vi "_emi_ SMLoop Error Check.vi"(0 "Loop Index":u16, 1 "Command ID":T1, 7 "Loop  Current Error State":errorcluster, 9 "Current Loop Error/Warning Source":enum16{"No Error", "Start", "Normal", "Stop"}(ring), 11 "Error in":errorcluster) -> (4 "Loop Index out":u16, 8 "Loop Error state out":errorcluster, 10 "Source Out":enum16{"No Error", "Start", "Normal", "Stop"}(ring), 15 "error out":errorcluster)   [LabVIEW 2011]
uses:
  _emi_ SMLoop sates.ctl
  emi_Read System ID.vi
  Private/_emi_GFV System ID.vi
  <vilib>/Utility/error.llb/Clear Errors.vi
  S&E reporting/Private/_emi_S&E Q Generator.vi
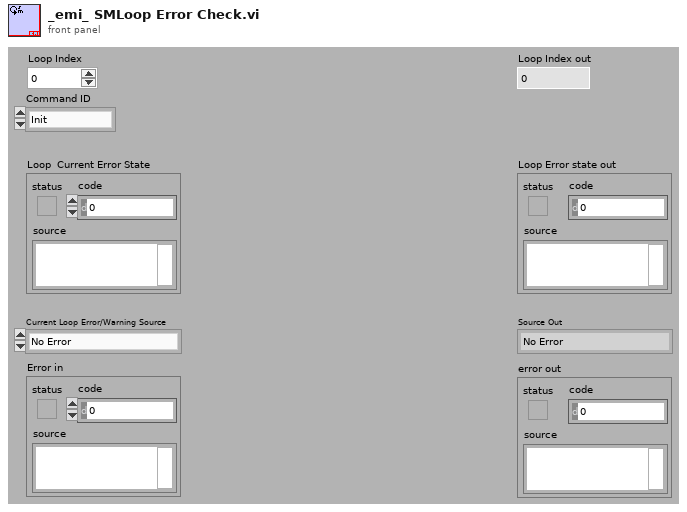
[diagram p1: front panel]
types:
  T1 = typedef "_emi_ SMLoop sates.ctl" = enum16{"Init", "Standby", "Start", "Normal Operation", "Stop", "Error Handling", "End", "Post"}
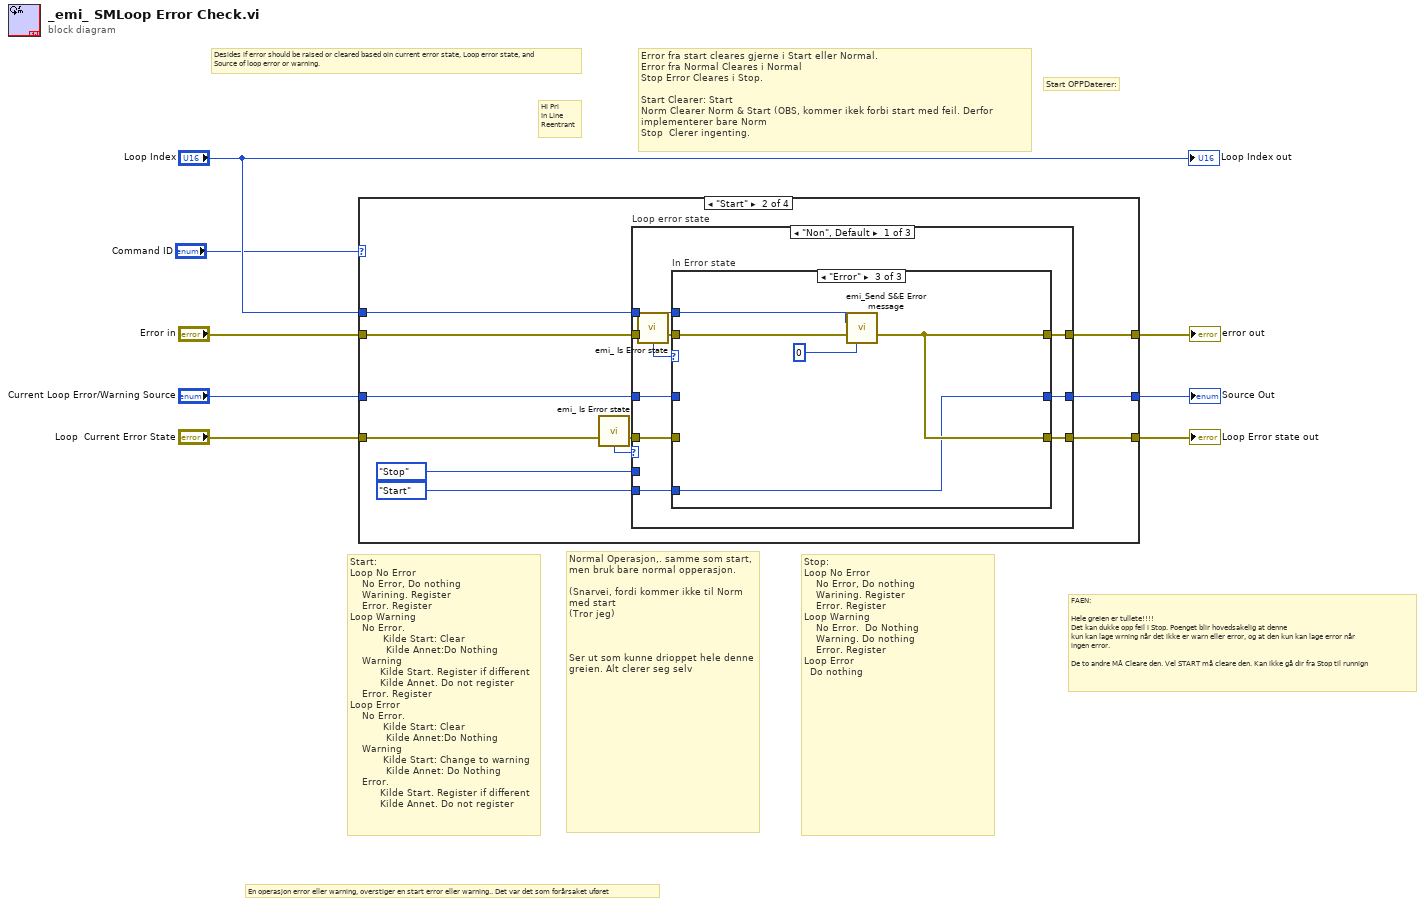
[diagram p0: block diagram]
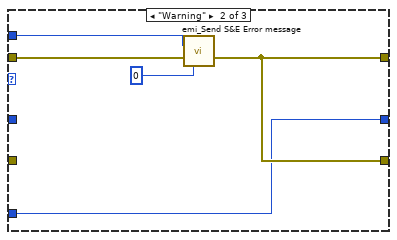
[diagram p4: hidden frame]
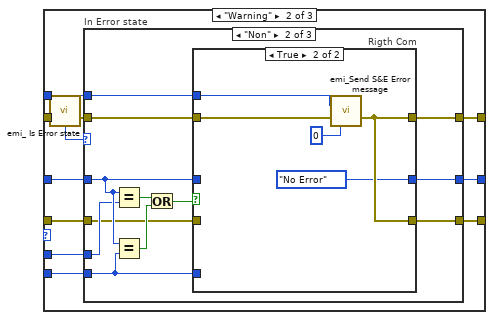
[diagram p5: hidden frame]
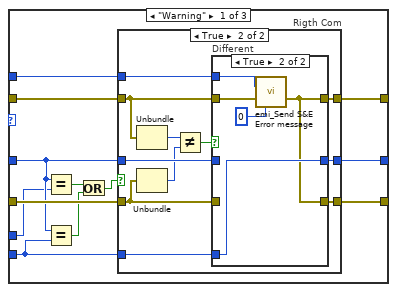
[diagram p6: hidden frame]
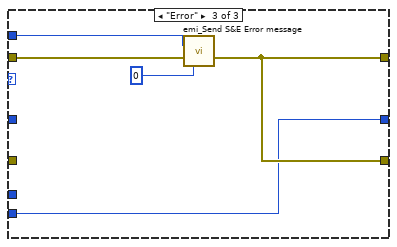
[diagram p10: hidden frame]
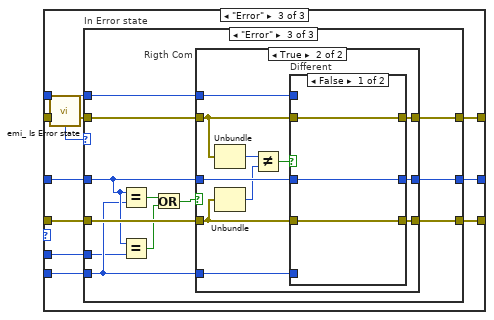
[diagram p11: hidden frame]
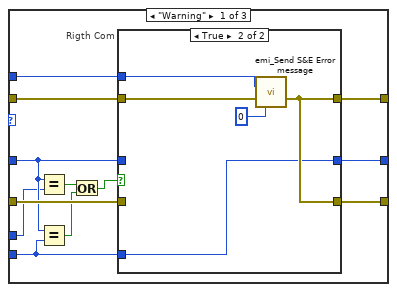
[diagram p12: hidden frame]
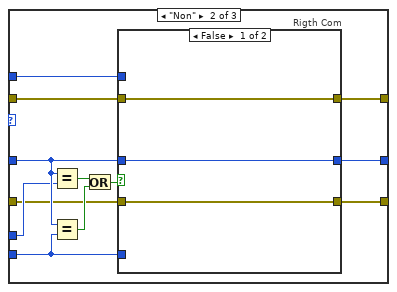
[diagram p14: hidden frame]
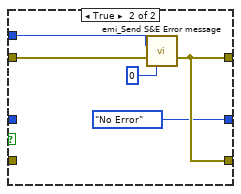
[diagram p15: hidden frame]
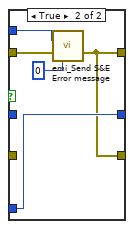
[diagram p17: hidden frame]
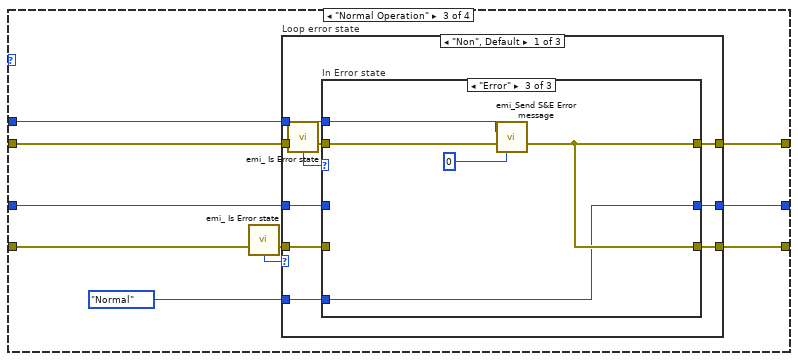
[diagram p18: hidden frame]
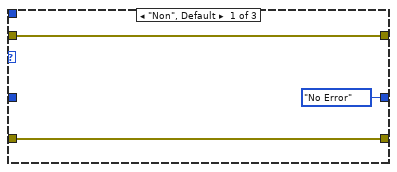
[diagram p19: hidden frame]
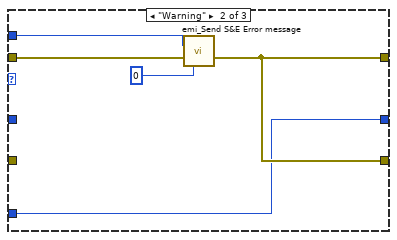
[diagram p20: hidden frame]
diagram:
  # "FAEN:\n\nHele greien er tullete!!!!\nDet kan dukke opp feil i Stop. Poenget blir hovedsakelig at denne\nkun kan lage wrning når det ikke er warn eller error, og at den kun kan lage error når\ningen error.\n\nDe to andre MÅ Cleare den. Vel START må cleare den. Kan ikke gå dir fra Stop til runnign"
  # "Stop:\nLoop No Error          \n    No Error, Do nothing\n    Warining. Register\n    Error. Register\nLoop Warning\n    No Error.  Do Nothing\n    Warning. Do nothing\n    Error. Register\nLoop Error\n  Do nothing"
  # "Normal Operasjon,. samme som start, men bruk bare normal opperasjon.\n\n(Snarvei, fordi kommer ikke til Norm med start\n(Tror jeg)\n\n\n\nSer ut som kunne drioppet hele denne greien. Alt clerer seg selv"
  # "En operasjon error eller warning, overstiger en start error eller warning.. Det var det som forårsaket uføret"
  # "Start OPPDaterer:"
  # "Start:\nLoop No Error          \n    No Error, Do nothing\n    Warining. Register\n    Error. Register\nLoop Warning\n    No Error. \n           Kilde Start: Clear\n            Kilde Annet:Do Nothing\n    Warning\n          Kilde Start. Register if different\n          Kilde Annet. Do not register\n    Error. Register\nLoop Error\n    No Error. \n           Kilde Start: Clear\n            Kilde Annet:Do Nothing\n    Warning\n           Kilde Start: Change to warning\n            Kilde Annet: Do Nothing\n    Error.\n          Kilde Start. Register if different\n          Kilde Annet. Do not register"
  # "Error fra start cleares gjerne i Start eller Normal.\nError fra Normal Cleares i Normal\nStop Error Cleares i Stop.\n\nStart Clearer: Start\nNorm Clearer Norm & Start (OBS, kommer ikek forbi start med feil. Derfor implementerer bare Norm\nStop  Clerer ingenting."
  # "Desides if error should be raised or cleared based oin current error state, Loop error state, and \nSource of loop error or warning."
  # "Hi Pri \nIn Line \nReentrant"
  n1 = case shown="\"Start\"" "Command ID" {
    tunnel: "Loop  Current Error State" -> [w9 w18 w206 w317]
    tunnel: [w9 w22 w210 w321] -> w7
    tunnel: [w10 w21 w209 w320] -> w6
    tunnel: "Current Loop Error/Warning Source" -> [w10 w13 w201 w312]
    tunnel: [w11 w20 w208 w319] -> w4
    tunnel: "Error in" -> [w11 w15 w203 w314]
    tunnel: "Loop Index" -> [_ w19 w207 w318]
    frame "Init", Default {
    }
    frame "Start" {
      n2 = call "emi_ Is Error state.vi"("error in (no error)"=w18) -> ("error out"=w17:errorcluster, "Error State"=w16:enum16{"Non", "Warning", "Error"})  [unwired: 13 in]
      n3 = case "Loop error state" shown="\"Non\", Default" w16 {
        tunnel: w19 -> [w32 w56 w126]
        tunnel: [w31 w55 w125] -> w20
        tunnel: w13 -> [w29 w53 w123]
        tunnel: [w30 w54 w124] -> w21
        tunnel: [w28 w52 w122] -> w22
        tunnel: w17 -> [w27 w51 w121]
        tunnel: w15 -> [w26 w50 w120]
        tunnel: enum16{"No Error", "Start", "Normal", "Stop"}."Start" ("Error source") -> [w23 w47 w117]
        tunnel: enum16{"No Error", "Start", "Normal", "Stop"}."Stop" ("Error source") -> [_ w46 w116]
        frame "Non", Default {
          n4 = call "emi_ Is Error state.vi"("error in (no error)"=w26) -> ("error out"=w25:errorcluster, "Error State"=w24:enum16{"Non", "Warning", "Error"})  [unwired: 13 in]
          n5 = case "In Error state" shown="\"Error\"" w24 {
            tunnel: w32 -> [_ w40 w45]
            tunnel: [w34 w37 w42] -> w31
            tunnel: w25 -> [w34 w38 w43]
            tunnel: [w35 w36 w41] -> w30
            tunnel: w29 -> [w35 _ _]
            tunnel: [w33 w37 w42] -> w28
            tunnel: w27 -> [w33 _ _]
            tunnel: w23 -> [_ w36 w41]
            frame "Non", Default {
            }
            frame "Warning" {
              n6 = call "emi_Send S&E Error message.vi"("Loop ID in(No Loop)"=w40, "error in (no error)"=w38, "Var Index"=u16 0 ("Loc Sub ID")) -> ("error out"=w37:errorcluster)  [unwired: 11 in, 1 out]
            }
            frame "Error" {
              n7 = call "emi_Send S&E Error message.vi"("Loop ID in(No Loop)"=w45, "error in (no error)"=w43, "Var Index"=u16 0 ("Loc Sub ID")) -> ("error out"=w42:errorcluster)  [unwired: 11 in, 1 out]
            }
          }
        }
        frame "Warning" {
          n8 = call "emi_ Is Error state.vi"("error in (no error)"=w50) -> ("error out"=w49:errorcluster, "Error State"=w48:enum16{"Non", "Warning", "Error"})  [unwired: 13 in]
          n9 = case "In Error state" shown="\"Non\"" w48 {
            tunnel: w56 -> [w68 w102 w115]
            tunnel: [w67 w101 w112] -> w55
            tunnel: w49 -> [w64 w98 w113]
            tunnel: [w65 w99 w111] -> w54
            tunnel: w53 -> [w59 w94 _]
            tunnel: [w66 w100 w112] -> w52
            tunnel: w51 -> [w63 w91 _]
            tunnel: w47 -> [w58 w93 w111]
            tunnel: w46 -> [w57 w92 _]
            frame "Warning" {
              n10 = Equal?(x=w59, y=w57) -> (x = y?=w62:bool)
              n11 = Equal?(x=w59, y=w58) -> (x = y?=w61:bool)
              n12 = Or(x=w62, y=w61) -> (x .or. y?=w60:bool)
              n13 = case "Rigth Com" shown="True" w60 {
                tunnel: w68 -> [_ w82]
                tunnel: w64 -> [w70 w80]
                tunnel: [w70 w81] -> w67
                tunnel: [w71 w79] -> w66
                tunnel: [w69 w78] -> w65
                tunnel: w58 -> [_ w72]
                tunnel: w63 -> [w71 w76]
                tunnel: w59 -> [w69 w77]
                frame False {
                }
                frame True {
                  n14 = Unbundle(w80) -> ("code"=w75:i32)  [unwired: 2 out]
                  n15 = Unbundle(w76) -> ("code"=w74:i32)  [unwired: 2 out]
                  n16 = Not Equal?(x=w75, y=w74) -> (x != y?=w73:bool)
                  n17 = case "Different" shown="True" w73 {
                    tunnel: w82 -> [_ w90]
                    tunnel: w80 -> [w84 w88]
                    tunnel: [w84 w86] -> w81
                    tunnel: w76 -> [w85 _]
                    tunnel: [w85 w86] -> w79
                    tunnel: [w83 w87] -> w78
                    tunnel: w77 -> [w83 _]
                    tunnel: w72 -> [_ w87]
                    frame False {
                    }
                    frame True {
                      n18 = call "emi_Send S&E Error message.vi"("Loop ID in(No Loop)"=w90, "error in (no error)"=w88, "Var Index"=u16 0 ("Loc Sub ID")) -> ("error out"=w86:errorcluster)  [unwired: 11 in, 1 out]
                    }
                  }
                }
              }
            }
            frame "Non" {
              n19 = Equal?(x=w94, y=w92) -> (x = y?=w97:bool)
              n20 = Equal?(x=w94, y=w93) -> (x = y?=w96:bool)
              n21 = Or(x=w97, y=w96) -> (x .or. y?=w95:bool)
              n22 = case "Rigth Com" shown="True" w95 {
                tunnel: w102 -> [_ w110]
                tunnel: w98 -> [w104 w109]
                tunnel: [w104 w108] -> w101
                tunnel: [w105 w108] -> w100
                tunnel: [w103 enum16{"No Error", "Start", "Normal", "Stop"}."No Error" ("Current Loop Error/Warning Source")] -> w99
                tunnel: w93 -> [_ _]
                tunnel: w91 -> [w105 _]
                tunnel: w94 -> [w103 _]
                frame False {
                }
                frame True {
                  n23 = call "emi_Send S&E Error message.vi"("Loop ID in(No Loop)"=w110, "error in (no error)"=w109, "Var Index"=u16 0 ("Loc Sub ID")) -> ("error out"=w108:errorcluster)  [unwired: 11 in, 1 out]
                }
              }
            }
            frame "Error" {
              n24 = call "emi_Send S&E Error message.vi"("Loop ID in(No Loop)"=w115, "error in (no error)"=w113, "Var Index"=u16 0 ("Loc Sub ID")) -> ("error out"=w112:errorcluster)  [unwired: 11 in, 1 out]
            }
          }
        }
        frame "Error" {
          n25 = call "emi_ Is Error state.vi"("error in (no error)"=w120) -> ("error out"=w119:errorcluster, "Error State"=w118:enum16{"Non", "Warning", "Error"})  [unwired: 13 in]
          n26 = case "In Error state" shown="\"Error\"" w118 {
            tunnel: w126 -> [w138 w158 w177]
            tunnel: [w137 w157 w176] -> w125
            tunnel: w119 -> [w134 w154 w178]
            tunnel: [w135 w155 w174] -> w124
            tunnel: w123 -> [w129 w150 w169]
            tunnel: [w136 w156 w173] -> w122
            tunnel: w121 -> [w133 w147 w175]
            tunnel: w117 -> [w128 w149 w168]
            tunnel: w116 -> [w127 w148 w167]
            frame "Warning" {
              n27 = Equal?(x=w129, y=w127) -> (x = y?=w132:bool)
              n28 = Equal?(x=w129, y=w128) -> (x = y?=w131:bool)
              n29 = Or(x=w132, y=w131) -> (x .or. y?=w130:bool)
              n30 = case "Rigth Com" shown="True" w130 {
                tunnel: w138 -> [_ w146]
                tunnel: w134 -> [w140 w145]
                tunnel: [w140 w144] -> w137
                tunnel: [w141 w144] -> w136
                tunnel: [w139 w143] -> w135
                tunnel: w128 -> [_ w143]
                tunnel: w133 -> [w141 _]
                tunnel: w129 -> [w139 _]
                frame False {
                }
                frame True {
                  n31 = call "emi_Send S&E Error message.vi"("Loop ID in(No Loop)"=w146, "error in (no error)"=w145, "Var Index"=u16 0 ("Loc Sub ID")) -> ("error out"=w144:errorcluster)  [unwired: 11 in, 1 out]
                }
              }
            }
            frame "Non" {
              n32 = Equal?(x=w150, y=w148) -> (x = y?=w153:bool)
              n33 = Equal?(x=w150, y=w149) -> (x = y?=w152:bool)
              n34 = Or(x=w153, y=w152) -> (x .or. y?=w151:bool)
              n35 = case "Rigth Com" shown="False" w151 {
                tunnel: w158 -> [_ w166]
                tunnel: w154 -> [w160 w165]
                tunnel: [w160 w164] -> w157
                tunnel: [w161 w164] -> w156
                tunnel: [w159 enum16{"No Error", "Start", "Normal", "Stop"}."No Error" ("Current Loop Error/Warning Source")] -> w155
                tunnel: w149 -> [_ _]
                tunnel: w147 -> [w161 _]
                tunnel: w150 -> [w159 _]
                frame False {
                }
                frame True {
                  n36 = call "emi_Send S&E Error message.vi"("Loop ID in(No Loop)"=w166, "error in (no error)"=w165, "Var Index"=u16 0 ("Loc Sub ID")) -> ("error out"=w164:errorcluster)  [unwired: 11 in, 1 out]
                }
              }
            }
            frame "Error" {
              n37 = Equal?(x=w169, y=w168) -> (x = y?=w172:bool)
              n38 = Equal?(x=w169, y=w167) -> (x = y?=w171:bool)
              n39 = Or(x=w172, y=w171) -> (x .or. y?=w170:bool)
              n40 = case "Rigth Com" shown="True" w170 {
                tunnel: w177 -> [_ w192]
                tunnel: w178 -> [w180 w190]
                tunnel: [w180 w191] -> w176
                tunnel: [w181 w189] -> w173
                tunnel: [w179 w188] -> w174
                tunnel: w168 -> [_ w182]
                tunnel: w175 -> [w181 w186]
                tunnel: w169 -> [w179 w187]
                frame False {
                }
                frame True {
                  n41 = Unbundle(w190) -> ("code"=w185:i32)  [unwired: 2 out]
                  n42 = Unbundle(w186) -> ("code"=w184:i32)  [unwired: 2 out]
                  n43 = Not Equal?(x=w185, y=w184) -> (x != y?=w183:bool)
                  n44 = case "Different" shown="False" w183 {
                    tunnel: w192 -> [_ w200]
                    tunnel: w190 -> [w194 w198]
                    tunnel: [w194 w196] -> w191
                    tunnel: w186 -> [w195 _]
                    tunnel: [w195 w196] -> w189
                    tunnel: [w193 w197] -> w188
                    tunnel: w187 -> [w193 _]
                    tunnel: w182 -> [_ w197]
                    frame False {
                    }
                    frame True {
                      n45 = call "emi_Send S&E Error message.vi"("Loop ID in(No Loop)"=w200, "error in (no error)"=w198, "Var Index"=u16 0 ("Loc Sub ID")) -> ("error out"=w196:errorcluster)  [unwired: 11 in, 1 out]
                    }
                  }
                }
              }
            }
          }
        }
      }
    }
    frame "Normal Operation" {
      n46 = call "emi_ Is Error state.vi"("error in (no error)"=w206) -> ("error out"=w205:errorcluster, "Error State"=w204:enum16{"Non", "Warning", "Error"})  [unwired: 13 in]
      n47 = case "Loop error state" shown="\"Non\", Default" w204 {
        tunnel: w207 -> [w220 w243 w282]
        tunnel: [w219 w242 w281] -> w208
        tunnel: w201 -> [w217 w240 w279]
        tunnel: [w218 w241 w280] -> w209
        tunnel: [w216 w239 w278] -> w210
        tunnel: w205 -> [w215 w238 w277]
        tunnel: w203 -> [w214 w237 w276]
        tunnel: enum16{"No Error", "Start", "Normal", "Stop"}."Normal" ("Error source") -> [w211 w234 w273]
        frame "Non", Default {
          n48 = call "emi_ Is Error state.vi"("error in (no error)"=w214) -> ("error out"=w213:errorcluster, "Error State"=w212:enum16{"Non", "Warning", "Error"})  [unwired: 13 in]
          n49 = case "In Error state" shown="\"Error\"" w212 {
            tunnel: w220 -> [_ w228 w233]
            tunnel: [w223 w225 w230] -> w219
            tunnel: w213 -> [w223 w226 w231]
            tunnel: [enum16{"No Error", "Start", "Normal", "Stop"}."No Error" ("Error source") w224 w229] -> w218
            tunnel: w217 -> [_ _ _]
            tunnel: [w222 w225 w230] -> w216
            tunnel: w215 -> [w222 _ _]
            tunnel: w211 -> [_ w224 w229]
            frame "Non", Default {
            }
            frame "Warning" {
              n50 = call "emi_Send S&E Error message.vi"("Loop ID in(No Loop)"=w228, "error in (no error)"=w226, "Var Index"=u16 0 ("Loc Sub ID")) -> ("error out"=w225:errorcluster)  [unwired: 11 in, 1 out]
            }
            frame "Error" {
              n51 = call "emi_Send S&E Error message.vi"("Loop ID in(No Loop)"=w233, "error in (no error)"=w231, "Var Index"=u16 0 ("Loc Sub ID")) -> ("error out"=w230:errorcluster)  [unwired: 11 in, 1 out]
            }
          }
        }
        frame "Warning" {
          n52 = call "emi_ Is Error state.vi"("error in (no error)"=w237) -> ("error out"=w236:errorcluster, "Error State"=w235:enum16{"Non", "Warning", "Error"})  [unwired: 13 in]
          n53 = case "In Error state" shown="\"Warning\"" w235 {
            tunnel: w243 -> [w254 w267 w272]
            tunnel: [w253 w266 w269] -> w242
            tunnel: w236 -> [w249 w264 w270]
            tunnel: [w251 enum16{"No Error", "Start", "Normal", "Stop"}."No Error" ("Current Loop Error/Warning Source") w268] -> w241
            tunnel: w240 -> [w248 _ _]
            tunnel: [w252 w266 w269] -> w239
            tunnel: w238 -> [w247 _ _]
            tunnel: w234 -> [w250 _ w268]
            frame "Warning" {
              n54 = Unbundle(w249) -> ("code"=w246:i32)  [unwired: 2 out]
              n55 = Unbundle(w247) -> ("code"=w245:i32)  [unwired: 2 out]
              n56 = Not Equal?(x=w246, y=w245) -> (x != y?=w244:bool)
              n57 = case "Different" shown="True" w244 {
                tunnel: w254 -> [_ w262]
                tunnel: w249 -> [w256 w260]
                tunnel: [w256 w258] -> w253
                tunnel: w247 -> [w257 _]
                tunnel: [w257 w258] -> w252
                tunnel: [w255 w259] -> w251
                tunnel: w248 -> [w255 _]
                tunnel: w250 -> [_ w259]
                frame False {
                }
                frame True {
                  n58 = call "emi_Send S&E Error message.vi"("Loop ID in(No Loop)"=w262, "error in (no error)"=w260, "Var Index"=u16 0 ("Loc Sub ID")) -> ("error out"=w258:errorcluster)  [unwired: 11 in, 1 out]
                }
              }
            }
            frame "Non" {
              n59 = call "emi_Send S&E Error message.vi"("Loop ID in(No Loop)"=w267, "error in (no error)"=w264, "Var Index"=u16 0 ("Loc Sub ID")) -> ("error out"=w266:errorcluster)  [unwired: 11 in, 1 out]
            }
            frame "Error" {
              n60 = call "emi_Send S&E Error message.vi"("Loop ID in(No Loop)"=w272, "error in (no error)"=w270, "Var Index"=u16 0 ("Loc Sub ID")) -> ("error out"=w269:errorcluster)  [unwired: 11 in, 1 out]
            }
          }
        }
        frame "Error" {
          n61 = call "emi_ Is Error state.vi"("error in (no error)"=w276) -> ("error out"=w275:errorcluster, "Error State"=w274:enum16{"Non", "Warning", "Error"})  [unwired: 13 in]
          n62 = case "In Error state" shown="\"Non\"" w274 {
            tunnel: w282 -> [w287 w292 w302]
            tunnel: [w286 w291 w301] -> w281
            tunnel: w275 -> [w285 w289 w303]
            tunnel: [w284 enum16{"No Error", "Start", "Normal", "Stop"}."No Error" ("Current Loop Error/Warning Source") w300] -> w280
            tunnel: w279 -> [_ _ w298]
            tunnel: [w286 w291 w299] -> w278
            tunnel: w277 -> [_ _ w296]
            tunnel: w273 -> [w284 _ w297]
            frame "Warning" {
              n63 = call "emi_Send S&E Error message.vi"("Loop ID in(No Loop)"=w287, "error in (no error)"=w285, "Var Index"=u16 0 ("Loc Sub ID")) -> ("error out"=w286:errorcluster)  [unwired: 11 in, 1 out]
            }
            frame "Non" {
              n64 = call "emi_Send S&E Error message.vi"("Loop ID in(No Loop)"=w292, "error in (no error)"=w289, "Var Index"=u16 0 ("Loc Sub ID")) -> ("error out"=w291:errorcluster)  [unwired: 11 in, 1 out]
            }
            frame "Error" {
              n65 = Unbundle(w303) -> ("code"=w295:i32)  [unwired: 2 out]
              n66 = Unbundle(w296) -> ("code"=w294:i32)  [unwired: 2 out]
              n67 = Not Equal?(x=w295, y=w294) -> (x != y?=w293:bool)
              n68 = case "Different" shown="True" w293 {
                tunnel: w302 -> [_ w311]
                tunnel: w303 -> [w305 w309]
                tunnel: [w305 w307] -> w301
                tunnel: w296 -> [w306 _]
                tunnel: [w306 w307] -> w299
                tunnel: [w304 w308] -> w300
                tunnel: w298 -> [w304 _]
                tunnel: w297 -> [_ w308]
                frame False {
                }
                frame True {
                  n69 = call "emi_Send S&E Error message.vi"("Loop ID in(No Loop)"=w311, "error in (no error)"=w309, "Var Index"=u16 0 ("Loc Sub ID")) -> ("error out"=w307:errorcluster)  [unwired: 11 in, 1 out]
                }
              }
            }
          }
        }
      }
    }
    frame "Stop" {
      n70 = call "emi_ Is Error state.vi"("error in (no error)"=w317) -> ("error out"=w316:errorcluster, "Error State"=w315:enum16{"Non", "Warning", "Error"})  [unwired: 13 in]
      n71 = case "Loop error state" shown="\"Warning\"" w315 {
        tunnel: w318 -> [w331 w354 _]
        tunnel: [w330 w353 w368] -> w319
        tunnel: w312 -> [w328 w351 w367]
        tunnel: [w329 w352 w367] -> w320
        tunnel: [w327 w350 w366] -> w321
        tunnel: w316 -> [w326 w349 w366]
        tunnel: w314 -> [w325 w348 w368]
        tunnel: enum16{"No Error", "Start", "Normal", "Stop"}."Stop" ("Error source") -> [w322 w345 _]
        frame "Non", Default {
          n72 = call "emi_ Is Error state.vi"("error in (no error)"=w325) -> ("error out"=w324:errorcluster, "Error State"=w323:enum16{"Non", "Warning", "Error"})  [unwired: 13 in]
          n73 = case "In Error state" shown="\"Error\"" w323 {
            tunnel: w331 -> [_ w339 w344]
            tunnel: [w333 w336 w341] -> w330
            tunnel: w324 -> [w333 w337 w342]
            tunnel: [w334 w335 w340] -> w329
            tunnel: w328 -> [w334 _ _]
            tunnel: [w332 w336 w341] -> w327
            tunnel: w326 -> [w332 _ _]
            tunnel: w322 -> [_ w335 w340]
            frame "Non", Default {
            }
            frame "Warning" {
              n74 = call "emi_Send S&E Error message.vi"("Loop ID in(No Loop)"=w339, "error in (no error)"=w337, "Var Index"=u16 0 ("Loc Sub ID")) -> ("error out"=w336:errorcluster)  [unwired: 11 in, 1 out]
            }
            frame "Error" {
              n75 = call "emi_Send S&E Error message.vi"("Loop ID in(No Loop)"=w344, "error in (no error)"=w342, "Var Index"=u16 0 ("Loc Sub ID")) -> ("error out"=w341:errorcluster)  [unwired: 11 in, 1 out]
            }
          }
        }
        frame "Warning" {
          n76 = call "emi_ Is Error state.vi"("error in (no error)"=w348) -> ("error out"=w347:errorcluster, "Error State"=w346:enum16{"Non", "Warning", "Error"})  [unwired: 13 in]
          n77 = case "In Error state" shown="\"Error\"" w346 {
            tunnel: w354 -> [_ _ w365]
            tunnel: [w357 w359 w362] -> w353
            tunnel: w347 -> [w357 w359 w363]
            tunnel: [w356 w360 w361] -> w352
            tunnel: w351 -> [w356 w360 _]
            tunnel: [w355 w358 w362] -> w350
            tunnel: w349 -> [w355 w358 _]
            tunnel: w345 -> [_ _ w361]
            frame "Warning" {
            }
            frame "Non" {
            }
            frame "Error" {
              n78 = call "emi_Send S&E Error message.vi"("Loop ID in(No Loop)"=w365, "error in (no error)"=w363, "Var Index"=u16 0 ("Loc Sub ID")) -> ("error out"=w362:errorcluster)  [unwired: 11 in, 1 out]
            }
          }
        }
        frame "Error" {
        }
      }
    }
  }
  "Loop Error state out" <- w7
  "Source Out" <- w6
  "error out" <- w4
  "Loop Index out" <- "Loop Index"
